vi "Merge Error.vi"(10 "Error":errorcluster, 11 "Base Queue in":refnum<class "Base Queue.lvclass">) -> (3 "Base Queue out":refnum<class "Base Queue.lvclass">)   [LabVIEW 2021, in "jettl.lvlib" / "Base Queue.lvlib" / "Base Queue.lvclass"]
uses:
  Base Queue.lvclass
  Base Queue.lvclass/Base Queue.ctl
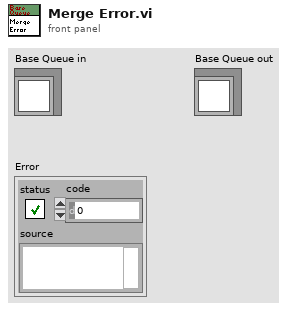
[diagram p1: front panel]
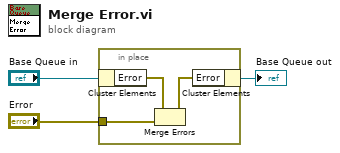
[diagram p0: block diagram]
diagram:
  n1 = in-place {
    in-place-border: "Error" -> [w4]
    n2 = in-place-cluster #1("Base Queue in") -> ("Error"=w6:errorcluster)
    n3 = Merge Errors(w6, w4) -> (w5:errorcluster)
    n4 = in-place-cluster #1("Error"=w5) -> (→"Base Queue out":refnum<class "Base Queue.lvclass">)
  }
